vi "Read State.vi"(8 "error in (no error)":errorcluster, 11 "B Context State in":refnum<class "B Context State.lvclass">) -> (0 "error out":errorcluster, 2 "State":refnum<class "State Pattern.lvclass">, 3 "B Context State out":refnum<class "B Context State.lvclass">)   [LabVIEW 2021, in "Context Actor.lvlib" / "B Context State.lvclass"]
uses:
  B Context State.lvclass
  State Pattern/State Pattern.lvclass
  B Context State.lvclass/B Context State.ctl
  Context Actor.lvclass
  C:/PPLs/Design-Patterns/State Pattern/State Pattern/State Pattern.lvclass
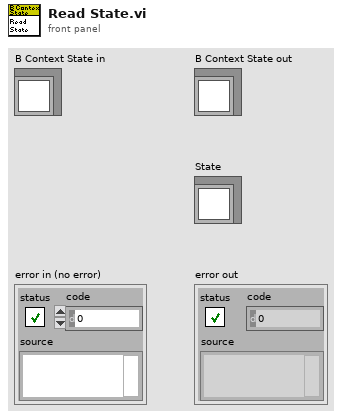
[diagram p1: front panel]
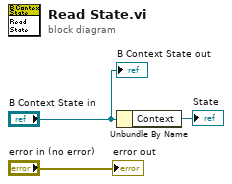
[diagram p0: block diagram]
diagram:
  n1 = Unbundle By Name("B Context State in") -> ("Context"=→"State":refnum<class "Context Actor.lvclass">)
  "error out" <- "error in (no error)"
  "B Context State out" <- "B Context State in"
